vi "SENS_BAND_BWID_TRAC.vi"(0 "VISA IN":refnum<visa-resource-name>, 1 "Track ON/OFF":bool, 5 "error in":errorcluster, 7 "Channel":i32=1) -> (14 "VISA Out":refnum<visa-resource-name>, 19 "error out":errorcluster)   [LabVIEW 2018, in "PNA-X.lvlib"]
doc: "SENSe<cnum>:BANDwidth | BWIDth:TRACk <bool> \n1621\n\n(Read-Write) Sets and returns the state of the Reduce IF BW at Low Frequencies feature. \n(Use either Sense:Bandwidth:Track or Sense:Bwidth:Track). \nParameters \n<cnum> Any existing channel number. If unspecified, value is set to 1 \n<bool> Choose from: \nON or 1 - Reduce IF BW at Low Frequencies is set ON \nOFF or 0 - Reduce IF BW at Low Frequencies is set OFF \nExamples SENS:BWID:TRAC OFF \nsense2:bandwidth:track 1 \nQuery Syntax SENSe<cnum>:BANDwidth | BWIDth:TRACk? \nReturn Type Boolean \nDefault ON \n1622\n\nSense:Correction Commands \nPerforms and applies calibration and other error correction features. \nTo perform Guided Calibration, see Sens:Corr Coll:GUIDed. \n1623\n\nClick on a blue keyword to view the command details. \nSee Also \nExample Programs \nNew See Calibrating the PNA Using SCPI \nLearn about Measurement Calibration \nSynchronizing the PNA and Controller \nSCPI Command Tree"
uses:
  PNA-X.lvlib
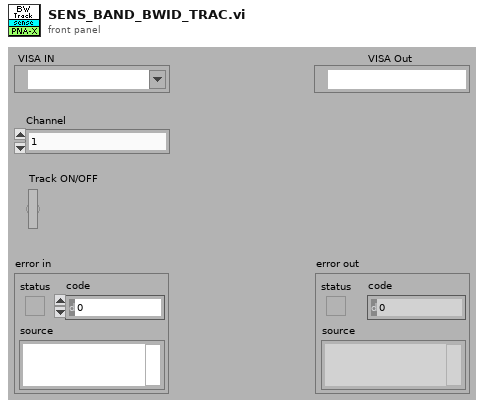
[diagram p1: front panel]
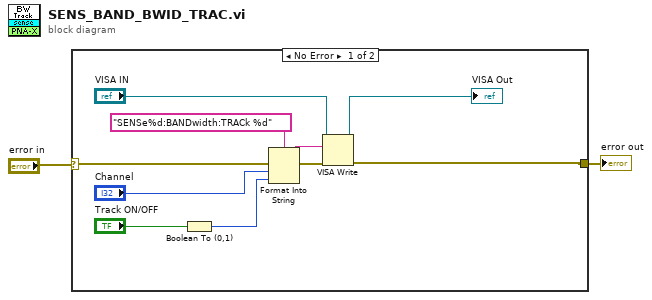
[diagram p0: block diagram]
diagram:
  n1 = case shown="No Error" "error in" {
    selector: "error in" -> [w12 w13]
    tunnel: [w7 w13] -> w1
    frame No Error {
      n2 = Boolean To (0,1)(Boolean="Track ON/OFF") -> (0, 1=w3:i16)
      n3 = Format Into String(format string="SENSe%d:BANDwidth:TRACk %d" ("Cmdline"), error in=w12, "Channel", w3) -> (resulting string=w10:string, error out=w11:errorcluster)  [unwired: 1 in]
      n4 = VISA Write(VISA resource name="VISA IN", write buffer=w10, error in (no error)=w11) -> (VISA resource name out=→"VISA Out":refnum<visa-resource-name>, error out=w7:errorcluster)  [unwired: 1 out]
    }
    frame Error {
    }
  }
  "error out" <- w1
